vi "Elevator Controller.vi"(8 "error in":errorcluster) -> ()   [LabVIEW 2018]
doc: "This VI executes continuously carrying out the current operation and responding to updates or new operations. It will often contain the timing or control code that is difficult to place directly in TeleOp. This VI generally opens all sensors and motors and isolates the rest of the robot code from knowing how the operations are carried out."
uses:
  Elevator Setpoints.ctl
  Elevator Operations.ctl
  <vilib>/Rock Robotics/WPI/ThirdParty/Phoenix-LabVIEW/Motor Controller/Controls/CTRE_Phoenix_MotorControl_NeutralMode.ctl
  <vilib>/Rock Robotics/WPI/ThirdParty/Phoenix-LabVIEW/Motor Controller/Controls/CTRE_Phoenix_MotorControl_ControlMode.ctl
  <vilib>/Rock Robotics/WPI/ThirdParty/Phoenix-LabVIEW/Motor Controller/Controls/CTRE_Phoenix_MotorControl_FeedbackDevice.ctl
  <vilib>/Rock Robotics/SystemInterfaces/DIO/FPGA_DIOChannel.ctl
  <vilib>/Rock Robotics/Network Tables/NT Write Boolean.vi
  <vilib>/Rock Robotics/WPI/ThirdParty/Phoenix-LabVIEW/Motor Controller/Get/CTRE_Phoenix_MotorController_GetQuadratureData.vi
  <vilib>/Rock Robotics/Network Tables/NT Write Number.vi
panel:
  out "Current\nCmd":string
  # "Tip: It may be helpful to observe inputs and sensor values.\nYou may also want to display tuning or debugging controls."
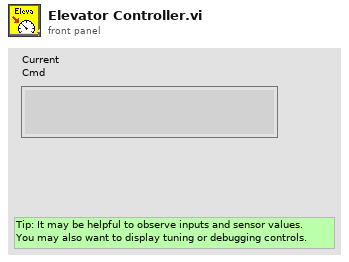
[diagram p1: front panel]
types:
  T1 = typedef "FPGA_DIOChannel.ctl" = enum8{"DIO 0", "DIO 1", "DIO 2", "DIO 3", "DIO 4", "DIO 5", "DIO 6", "DIO 7", "DIO 8", "DIO 9", "DIO MXP 0", "DIO MXP 1", "DIO MXP 2", "DIO MXP 3", "DIO MXP 4", "DIO MXP 5", "DIO MXP 6", "DIO MXP 7", "DIO MXP 8", "DIO MXP 9", "DIO MXP 10", "DIO MXP 11", "DIO MXP 12", "DIO MXP 13", "DIO MXP 14", "DIO MXP 15", "SPI Port CS1", "SPI Port CS2", "SPI Port CS3", "SPI Port MISO", "SPI Port MOSI", "Invalid"}
  T2 = typedef "CTRE_Phoenix_MotorControl_FeedbackDevice.ctl" = i8
  T3 = typedef "CTRE_Phoenix_MotorControl_ControlMode.ctl" = u16
  T4 = typedef "CTRE_Phoenix_MotorControl_NeutralMode.ctl" = enum8{"EEPROMSetting", "Override to Coast", "Override to Brake"}
  T5 = typedef "Elevator Setpoints.ctl" = cluster{"Operation":T6, "Setpoint":dbl, "Duration":dbl}
  T6 = typedef "Elevator Operations.ctl" = enum16{"Reserve", "Read Current", "Immediate", "Move Elevator", "Elevator Preset", "Elevator For Time"}
  T7 = typedef "WPI_MotorControlDeviceRef.ctl" = cluster{"DeviceStatus":errorcluster, "Type":T8, "PWM":cluster{"PWM Channel":T9, "DeadBand":T10}, "CAN":cluster{"Device Number":u8, "SetOutput VI Ref":variant, "GetOutput VI Ref":variant, "Enable VI Ref":variant, "Disable VI Ref":variant, "Data":variant}, "Invert":bool, "DIO PWM":cluster{"PWM \"Enable\" Channel":T9, "DIOChannel":T1, "PWM Rate":dbl}}
  T8 = typedef "WPI_MotorControlType.ctl" = enum16{"PWM", "CAN", "DIO PWM"}
  T9 = typedef "FPGA_DIOPWMChannel.ctl" = enum8{"PWM 0", "PWM 1", "PWM 2", "PWM 3", "PWM 4", "PWM 5", "PWM 6", "PWM 7", "PWM 8", "PWM 9", "PWM MXP 0", "PWM MXP 1", "PWM MXP 2", "PWM MXP 3", "PWM MXP 4", "PWM MXP 5", "PWM MXP 6", "PWM MXP 7", "PWM MXP 8", "PWM MXP 9", "Invalid"}
  T10 = typedef "WPI_PWMDeadband.ctl" = cluster{"Name":string, "maxPositivePwm":i32, "minPositivePwm":i32, "centerPwm":i32, "maxNegativePwm":i32, "minNegativePwm":i32, "angularRange":u16}
  T11 = typedef "Command Status Info.ctl" = cluster{"Name":string, "Status":T12, "notifier out":T13}
  T12 = typedef "Completion Status.ctl" = enum16{"Successful", "Aborted", "Incomplete"}
  T13 = typedef "Completion Notifier.ctl" = refnum<notifier>
  T14 = cluster{"Current Command":T5, "Command Timing":cluster{"Start Time (ms)":u32, "Iterations":i32}, "Command Arguments":cluster{"Command Info":T11, "Description":string, "Default Command":T5, "queue out":refnum<queue>, "Subsystem Name":string}}
  T15 = typedef "WPI_DigitalInputDevRef.ctl" = cluster{"DevStatus":errorcluster, "DIO Channel":T1}
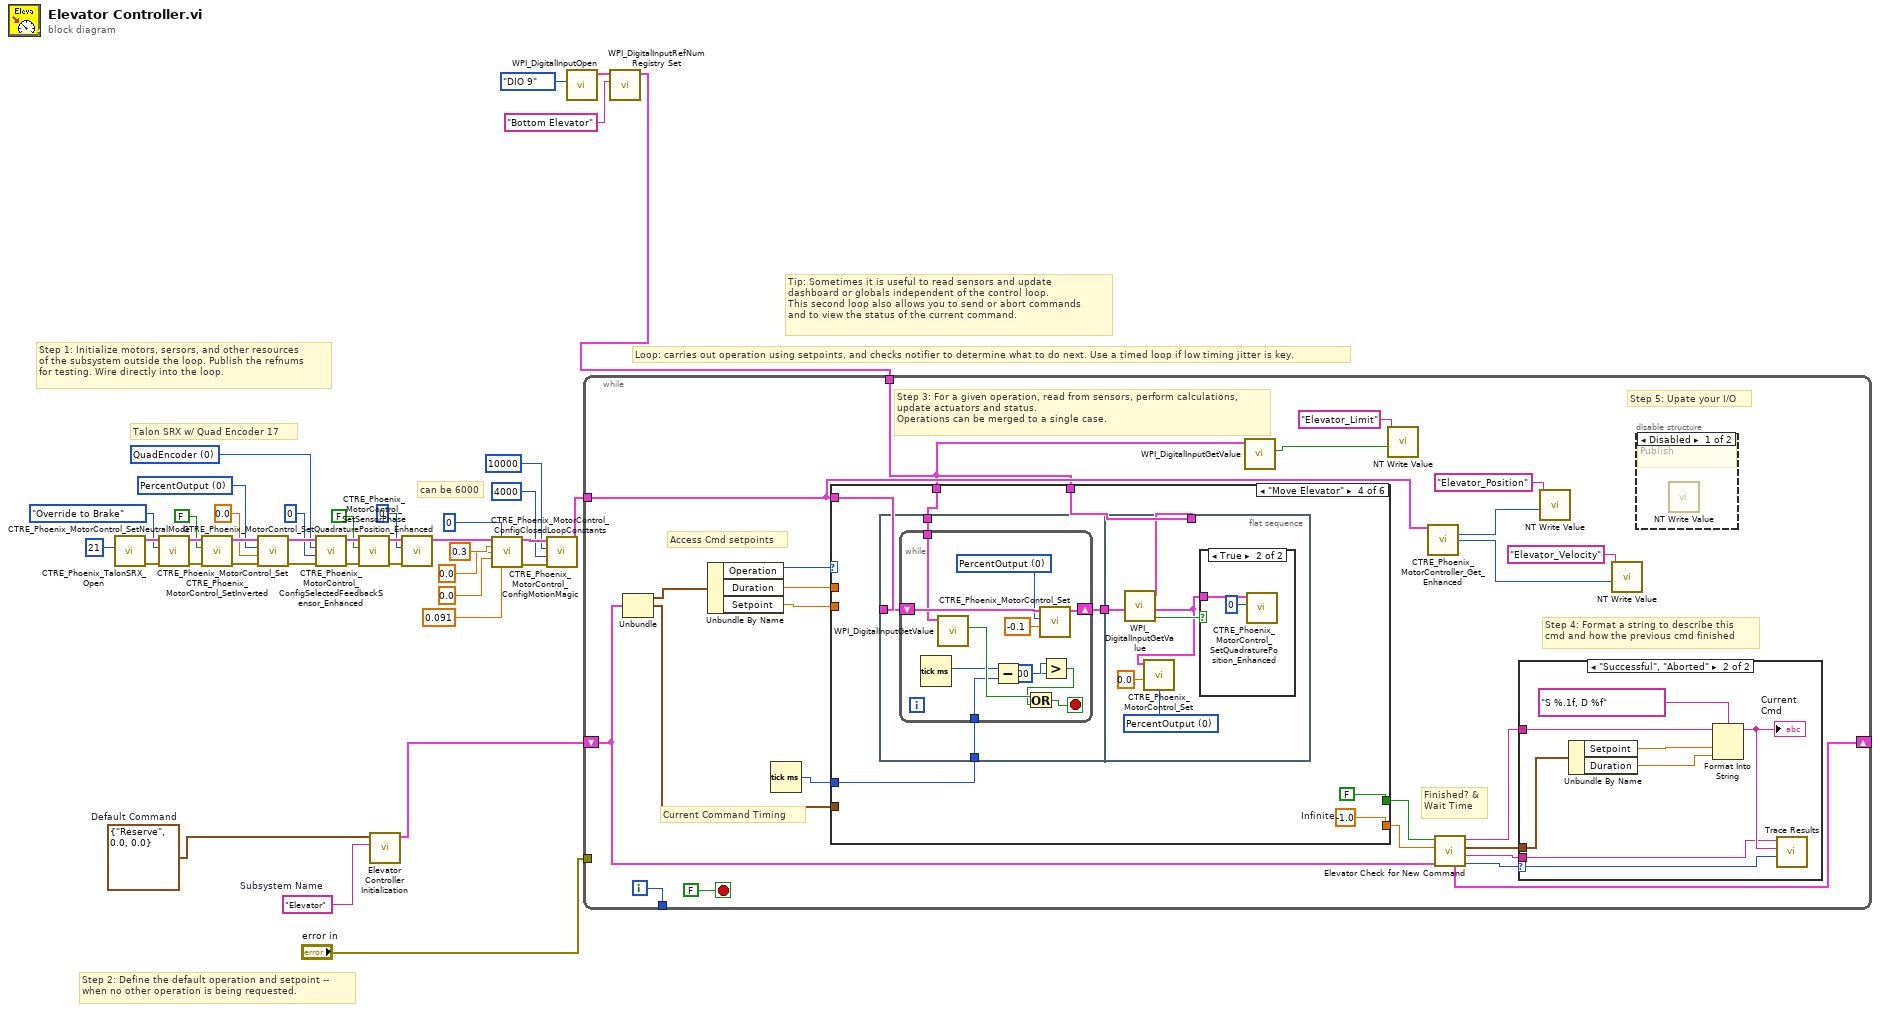
[diagram p0: block diagram]
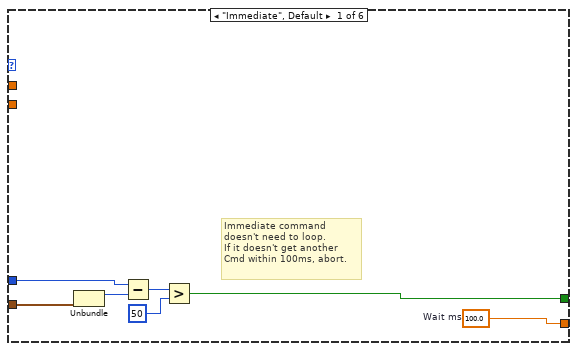
[diagram p4: hidden frame]
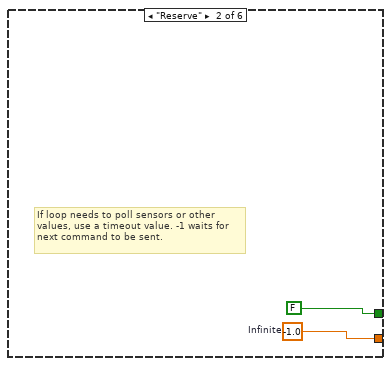
[diagram p5: hidden frame]
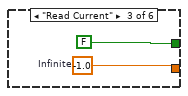
[diagram p6: hidden frame]
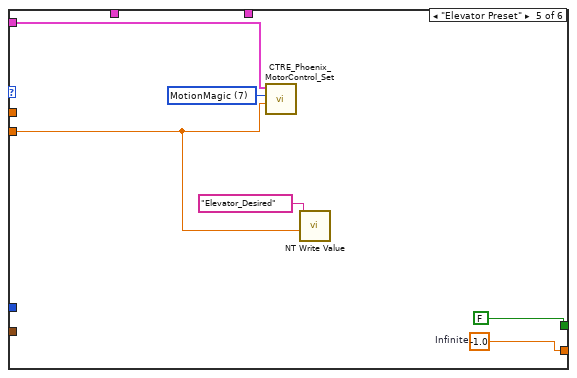
[diagram p8: hidden frame]
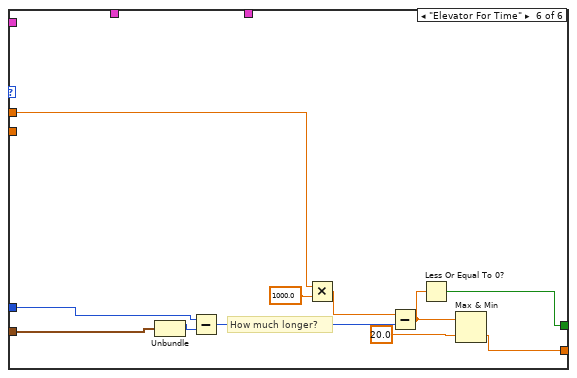
[diagram p9: hidden frame]
diagram:
  w19 = T2 0 items=["QuadEncoder"=0, "Analog"=2, "Tachometer"=4, "Pulse Width Encoded Position"=8, "Sensor Sum (S0 + S1)"=9, "Sensor Difference (D0 - D1)"=10, "Remote Source 0"=11, "Remote Source 1"=12, "Software Emulated"=15] ("Feedback Device")
  w21 = T3 0 items=["PercentOutput"=0, "Position"=1, "Velocity"=2, "Current"=3, "Follower"=5, "MotionProfile"=6, "MotionMagic"=7, "MotionProfileArc"=10, "Disabled"=15] ("Control Mode")
  w37 = T5 {"Operation"=enum."Reserve", "Setpoint"=0.0, "Duration"=0.0}  # Default Command
  w38 = "Elevator"  # Subsystem Name
  # "can be 6000"
  # "Talon SRX w/ Quad Encoder 17"
  # "Tip: Sometimes it is useful to read sensors and update\ndashboard or globals independent of the control loop.\nThis second loop also allows you to send or abort commands\nand to view the status of the current command."
  # "Step 2: Define the default operation and setpoint --\nwhen no other operation is being requested."
  # "Step 1: Initialize motors, sersors, and other resources\nof the subsystem outside the loop. Publish the refnums\nfor testing. Wire directly into the loop."
  # "Loop: carries out operation using setpoints, and checks notifier to determine what to do next. Use a timed loop if low timing jitter is key."
  n1 = call <vilib>:"CTRE_Phoenix_TalonSRX_Open.vi"("Device Number"=u8 21) -> ("error out"=w26:errorcluster, "CAN Talon SRX Ref"=w25:T7)  [unwired: 9 in]
  n2 = call <vilib>:"CTRE_Phoenix_MotorControl_SetNeutralMode.vi"("error in (no error)"=w26, "Motor Control Neutral Mode"=CTRE_Phoenix_MotorControl_NeutralMode."Override to Brake", "PhoenixMotorControlDevRef"=w25) -> ("error out"=w36:errorcluster, "PhoenixMotorControlDevRef"=w35:T7)  [unwired: 7 in]
  n3 = call <vilib>:"CTRE_Phoenix_MotorControl_SetInverted.vi"("error in (no error)"=w36, "Invert?"=FALSE, "PhoenixMotorControlDevRef"=w35) -> ("error out"=w34:errorcluster, "PhoenixMotorControlDevRef"=w33:T7)  [unwired: 7 in]
  n4 = call <vilib>:"CTRE_Phoenix_MotorControl_Set.vi"("error in (no error)"=w34, "Output"=0.0, "Control Mode"=w21, "PhoenixMotorControlDevRef"=w33) -> ("error out"=w27:errorcluster, "PhoenixMotorControlDevRef"=w32:T7)  [unwired: 6 in]
  n5 = call <vilib>:"CTRE_Phoenix_MotorControl_ConfigSelectedFeedbackSensor_Enhanced.vi"("error in (no error)"=w27, "pidLoopIdx"=0, "Feedback Device"=w19, "PhoenixMotorControlDevRef"=w32) -> ("error out"=w28:errorcluster, "PhoenixMotorControlDevRef"=w31:T7)  [unwired: 6 in]
  n6 = call <vilib>:"CTRE_Phoenix_MotorControl_SetSensorPhase.vi"("error in (no error)"=w28, "PhaseSensor"=FALSE, "PhoenixMotorControlDevRef"=w31) -> ("error out"=w29:errorcluster, "PhoenixMotorControlDevRef"=w30:T7)  [unwired: 7 in]
  n7 = call "Elevator Controller Initialization.vi"("Subsystem Name"=w38, "Default Command"=w37) -> ("Current Command"=w39:T14)  [unwired: 9 in]
  n8 = call <vilib>:"CTRE_Phoenix_MotorControl_SetQuadraturePosition_Enhanced.vi"("error in (no error)"=w29, "New Position"=0, "PhoenixMotorControlDevRef"=w30) -> ("PhoenixMotorControlDevRef"=w13:T7)  [unwired: 7 in, 1 out]
  n9 = call <vilib>:"CTRE_Phoenix_MotorControl_ConfigClosedLoopConstants.vi"("PhoenixMotorControlDevRef"=w13, "slotIdx"=0, "P"=0.3, "I"=0.0, "D"=0.0, "F"=0.091) -> ("PhoenixMotorControlDevRef"=w16:T7, "error out"=w17:errorcluster)  [unwired: 8 in]
  n10 = call <vilib>:"CTRE_Phoenix_MotorControl_ConfigMotionMagic.vi"("error in (no error)"=w17, "Acceleration"=4000, "Cruise Velocity"=10000, "PhoenixMotorControlDevRef"=w16) -> ("PhoenixMotorControlDevRef"=w5:T7)  [unwired: 6 in, 1 out]
  n11 = call <vilib>:"WPI_DigitalInputOpen.vi"("DIO Channel"=FPGA_DIOChannel."DIO 9") -> ("DigitalInputDevRef"=w3:T15)  [unwired: 9 in, 1 out]
  n12 = call <vilib>:"WPI_DigitalInputRefNum Registry Set.vi"("refnum name"="Bottom Elevator", "DigitalInputDevRef"=w3) -> ("DigitalInputDevRef"=w1:T15)  [unwired: 8 in, 1 out]
  n13 = while {
    shift-right: [w56] -> _
    shift-left: w39 -> [w49]
    tunnel: [w63] -> _
    tunnel: "error in" -> [_]
    tunnel: w5 -> [w48]
    tunnel: w1 -> [w41]
    i -> [w63]
    stop <- FALSE stop-if-true
    # "Step 5: Upate your I/O"
    # "Step 4: Format a string to describe this\ncmd and how the previous cmd finished"
    # "Current Command Timing"
    # "Access Cmd setpoints"
    # "Finished? &\nWait Time"
    # "Step 3: For a given operation, read from sensors, perform calculations,\nupdate actuators and status.\nOperations can be merged to a single case."
    n14 = Unbundle(w49) -> ("Current Command"=w62:T5, "Command Timing"=w58:cluster{"Start Time (ms)":u32, "Iterations":i32})  [unwired: 1 out]
    n15 = Unbundle By Name(w62) -> ("Operation"=w61:T6, "Duration"=w60:dbl, "Setpoint"=w57:dbl)
    n16 = Tick Count (ms)() -> (millisecond timer value=w59:u32)
    n17 = case shown="\"Move Elevator\"" w61 {
      tunnel: [w79 w81 w82 w89 w118 w122] -> w54
      tunnel: [w73 FALSE ("ignore previous (F)") FALSE ("ignore previous (F)") FALSE ("ignore previous (F)") FALSE ("ignore previous (F)") w121] -> w55
      tunnel: w58 -> [w75 _ _ _ _ w124]
      tunnel: w60 -> [_ _ _ _ _ w120]
      tunnel: w59 -> [w74 _ _ w87 _ w123]
      tunnel: w57 -> [_ _ _ _ w114 _]
      tunnel: w48 -> [_ _ _ w88 w116 _]
      tunnel: w41 -> [_ _ _ w86 _ _]
      tunnel: w41 -> [_ _ _ w84 _ _]
      frame "Immediate", Default {
        w79 = 100.0  # Wait ms
        # "Immediate command\ndoesn't need to loop.\nIf it doesn't get another\nCmd within 100ms, abort."
        n18 = Unbundle(w75) -> ("Start Time (ms)"=w78:u32)  [unwired: 1 out]
        n19 = Subtract(x=w74, y=w78) -> (x-y=w77:u32)
        n20 = Greater?(x=w77, y=u8 50 ("Left Motor")) -> (0:w73:bool)
      }
      frame "Reserve" {
        w81 = -1.0  # Infinite
        # "If loop needs to poll sensors or other\nvalues, use a timeout value. -1 waits for\nnext command to be sent."
      }
      frame "Read Current" {
        w82 = -1.0  # Infinite
      }
      frame "Move Elevator" {
        w89 = -1.0  # Infinite
        n21 = flat-sequence {
          tunnel: w88 -> [w94]
          tunnel: w87 -> [w92]
          tunnel: w86 -> [w91]
          tunnel: [w93] -> w85
          tunnel: w85 -> [w109]
          tunnel: w84 -> [w110]
          frame #0 {
            n22 = while {
              tunnel: w91 -> [w104]
              shift-right: [w103] -> w93
              shift-left: w94 -> [w106]
              tunnel: w92 -> [w99]
              stop <- w101 stop-if-true
              w105 = T3 0 items=["PercentOutput"=0, "Position"=1, "Velocity"=2, "Current"=3, "Follower"=5, "MotionProfile"=6, "MotionMagic"=7, "MotionProfileArc"=10, "Disabled"=15] ("Control Mode")
              n23 = Tick Count (ms)() -> (millisecond timer value=w98:u32)
              n24 = call <vilib>:"WPI_DigitalInputGetValue.vi"("DigitalInputDevRef"=w104) -> ("Value"=w100:bool)  [unwired: 8 in, 2 out]
              n25 = Subtract(x=w98, y=w99) -> (x-y=w97:u32)
              n26 = call <vilib>:"CTRE_Phoenix_MotorControl_Set.vi"("Output"=-0.1, "Control Mode"=w105, "PhoenixMotorControlDevRef"=w106) -> ("PhoenixMotorControlDevRef"=w103:T7)  [unwired: 7 in, 1 out]
              n27 = Greater?(x=w97, y=u32 2000) -> (0:w95:bool)
              n28 = Or(x=w100, y=w95) -> (x .or. y?=w101:bool)
            }
          }
          frame #1 {
            w108 = T3 0 items=["PercentOutput"=0, "Position"=1, "Velocity"=2, "Current"=3, "Follower"=5, "MotionProfile"=6, "MotionMagic"=7, "MotionProfileArc"=10, "Disabled"=15] ("Control Mode")
            n29 = call <vilib>:"WPI_DigitalInputGetValue.vi"("DigitalInputDevRef"=w110) -> ("Value"=w111:bool)  [unwired: 8 in, 2 out]
            n30 = call <vilib>:"CTRE_Phoenix_MotorControl_Set.vi"("Output"=0.0, "Control Mode"=w108, "PhoenixMotorControlDevRef"=w109) -> ()  [unwired: 7 in, 2 out]
            n31 = case shown="True" w111 {
              tunnel: w109 -> [_ w113]
              frame False {
              }
              frame True {
                n32 = call <vilib>:"CTRE_Phoenix_MotorControl_SetQuadraturePosition_Enhanced.vi"("New Position"=0, "PhoenixMotorControlDevRef"=w113) -> ()  [unwired: 8 in, 2 out]
              }
            }
          }
        }
      }
      frame "Elevator Preset" {
        w117 = T3 7 items=["PercentOutput"=0, "Position"=1, "Velocity"=2, "Current"=3, "Follower"=5, "MotionProfile"=6, "MotionMagic"=7, "MotionProfileArc"=10, "Disabled"=15] ("Control Mode")
        w118 = -1.0  # Infinite
        n33 = call <vilib>:"CTRE_Phoenix_MotorControl_Set.vi"("Output"=w114, "Control Mode"=w117, "PhoenixMotorControlDevRef"=w116) -> ()  [unwired: 7 in, 2 out]
        n34 = call-poly <vilib>:"NT Write Value.vi"("Numeric"=w114, "Name"="Elevator_Desired") -> ()  [unwired: 9 in, 1 out]
      }
      frame "Elevator For Time" {
        # "How much longer?"
        n35 = Unbundle(w124) -> ("Start Time (ms)"=w128:u32)  [unwired: 1 out]
        n36 = Subtract(x=w123, y=w128) -> (x-y=w130:u32)
        n37 = Multiply(x=w120, y=1000.0) -> (x*y=w125:dbl)
        n38 = Subtract(x=w125, y=w130) -> (x-y=w127:dbl)
        n39 = Less Or Equal To 0?(x=w127) -> (x <= 0?=w121:bool)
        n40 = Max & Min(x=w127, y=20.0) -> (min(x,y)=w122:dbl)  [unwired: 1 out]
      }
    }
    n41 = call <vilib>:"WPI_DigitalInputGetValue.vi"("DigitalInputDevRef"=w41) -> ("Value"=w42:bool)  [unwired: 8 in, 2 out]
    n42 = call-poly <vilib>:"NT Write Value.vi"("Boolean"=w42, "Name"="Elevator_Limit") -> ()  [unwired: 9 in, 1 out]
    n43 = call-poly <vilib>:"CTRE_Phoenix_MotorController_Get_Enhanced.vi"("PhoenixMotorControlDevRef"=w48) -> ("Quadrature Position"=w47:i32, "Quadrature Velocity"=w44:i32)  [unwired: 11 in, 2 out]
    n44 = call "Elevator Check for New Command.vi"("Current Command"=w49, "Wait time (ms)"=w54, "Finished?"=w55) -> ("Completion"=w50:T12, "Subsystem Name"=w51:string, "Current Command"=w52:T5, "Initial Trace String"=w53:string, "NextCommand"=w56:T14)  [unwired: 4 in]
    n45 = case shown="\"Successful\", \"Aborted\"" w50 {
      selector: w50 -> [_ w72]
      tunnel: w53 -> [_ w68]
      tunnel: w52 -> [_ w69]
      tunnel: w51 -> [_ w65]
      frame "Incomplete", Default {
        # "Continuing current command"
      }
      frame "Successful", "Aborted" {
        # "Report and setup for next command"
        n46 = Unbundle By Name(w69) -> ("Setpoint"=w71:dbl, "Duration"=w66:dbl)
        n47 = Format Into String(format string="S %.1f, D %f", initial string=w68, w71, w66) -> (resulting string=w67:string)  [unwired: 1 in, 1 out]
        "Current\nCmd" <- w67
        n48 = call <vilib>:"Trace Results.vi"("Status of previous command"=w72, "Description"=w67, "Subsystem"=w65) -> ()  [unwired: 9 in]
      }
    }
    n49 = call-poly <vilib>:"NT Write Value.vi"("Numeric"=w47, "Name"="Elevator_Position") -> ()  [unwired: 9 in, 1 out]
    n50 = call-poly <vilib>:"NT Write Value.vi"("Numeric"=w44, "Name"="Elevator_Velocity") -> ()  [unwired: 9 in, 1 out]
    n51 = disable-structure shown="Disabled" {
      frame Disabled {
        # "Publish"
        n52 = call-poly <vilib>:"NT Write Value.vi"() -> ()  [unwired: 11 in, 1 out]
      }
      frame Enabled {
      }
    }
  }
